vi "Write to config.vi"(0 "Insert name":T1(ring), 5 "File Name":string="Lifter config", 7 "Bottom":dbl format="%#_3g", 9 "Middle":dbl, 11 "Top":dbl) -> ()   [LabVIEW 2019]
uses:
  <vilib>/Utility/config.llb/Write Key (Double).vi
  <vilib>/Utility/config.llb/NI_LVConfig.lvlib
panel:
  out "appended path":path
  out "concatenated string":string
  out "error out":errorcluster
  in  "error in (no error)":errorcluster
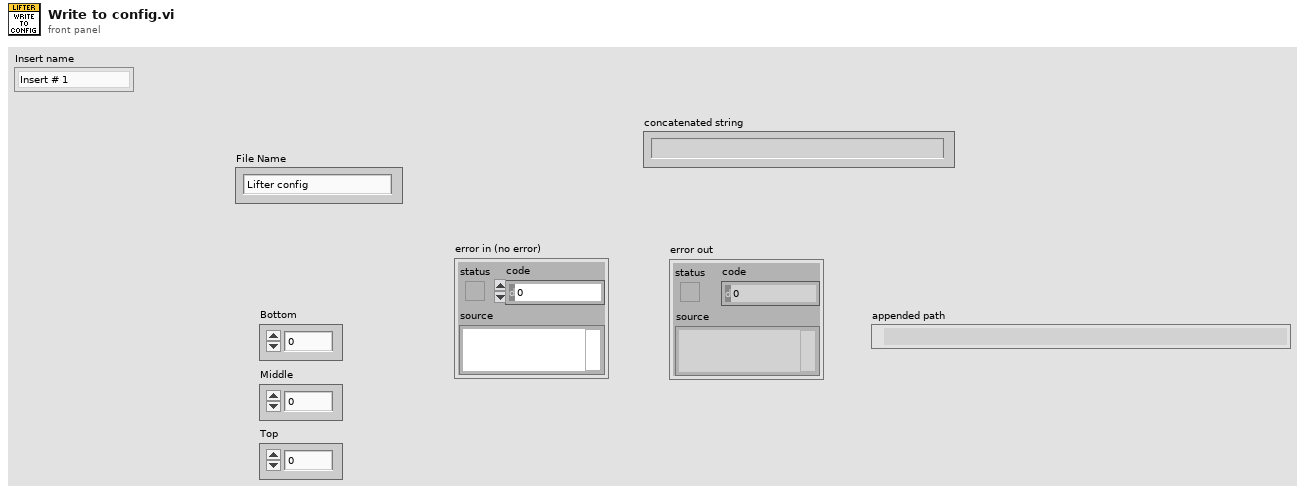
[diagram p1: front panel]
types:
  T1 = enum16{"Insert # 1", "Insert #2", "Calib insert"}
  T2 = typedef "NI_LVConfig.lvlib/Config Data RefNum.ctl" = refnum<k1>
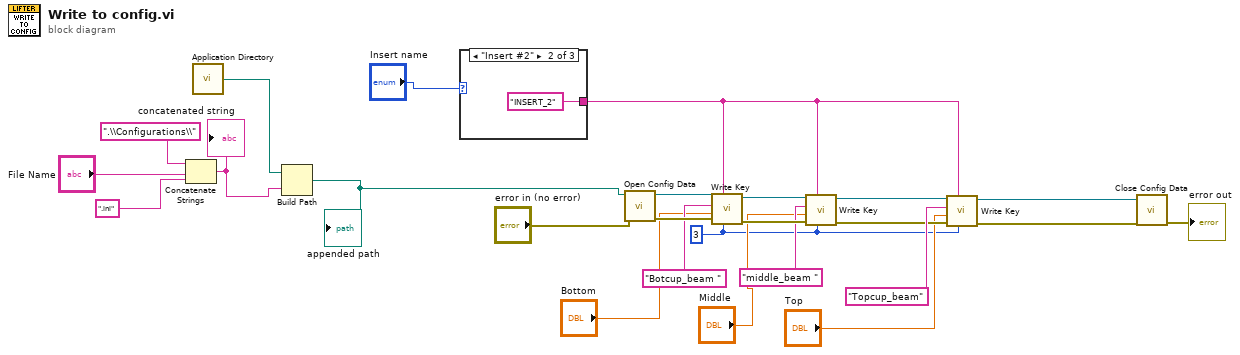
[diagram p0: block diagram]
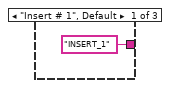
[diagram p2: hidden frame]
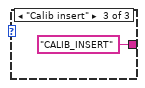
[diagram p3: hidden frame]
diagram:
  w3 = i16 3 ("precision (6)")
  n1 = Concatenate Strings(".\\Configurations\\" ("string"), "File Name", ".ini" ("string")) -> (w15:string)
  "concatenated string" <- w15
  n2 = call <vilib>:"Application Directory.vi"() -> ("Application Directory"=w13:path)
  n3 = Build Path(base path=w13, name or relative path=w15) -> (appended path=w10:path)
  "appended path" <- w10
  n4 = case shown="\"Insert #2\"" "Insert name" {
    tunnel: ["INSERT_1" ("section") "INSERT_2" ("section") "CALIB_INSERT" ("section")] -> w1
    frame "Insert # 1", Default {
    }
    frame "Insert #2" {
    }
    frame "Calib insert" {
    }
  }
  n5 = call <vilib>:"Open Config Data.vi"("error in (no error)"="error in (no error)", "configuration file path"=w10) -> ("error out"=w22:errorcluster, "refnum"=w25:T2)  [unwired: 7 in, 1 out]
  n6 = call-poly <vilib>:"Write Key.vi"("precision (6)"=w3, "section"=w1, "error in (no error)"=w22, "value"="Bottom", "key"="Botcup_beam ", "refnum"=w25) -> ("error out"=w23:errorcluster, "refnum out"=w24:T2)  [unwired: 3 in, 1 out]
  n7 = call-poly <vilib>:"Write Key.vi"("precision (6)"=w3, "section"=w1, "error in (no error)"=w23, "value"="Middle", "key"="middle_beam ", "refnum"=w24) -> ("error out"=w8:errorcluster, "refnum out"=w7:T2)  [unwired: 3 in, 1 out]
  n8 = call-poly <vilib>:"Write Key.vi"("precision (6)"=w3, "section"=w1, "error in (no error)"=w8, "value"="Top", "key"="Topcup_beam", "refnum"=w7) -> ("error out"=w5:errorcluster, "refnum out"=w4:T2)  [unwired: 3 in, 1 out]
  n9 = call <vilib>:"Close Config Data.vi"("error in (no error)"=w5, "refnum"=w4) -> ("error out"=→"error out":errorcluster)  [unwired: 8 in, 1 out]
